vi "Fitness Core Override.vi"(8 "error in (no error)":errorcluster, 9 "Target Binary String (LSb[0] - MSb[n-1])":bool[](array[boolean]), 10 "Parent Binary String (LSb[0] - MSb[n-1])":bool[](array[boolean]), 11 "Sentence in":refnum<class "Sentence.lvclass">) -> (0 "error out":errorcluster, 2 "Fitness Score":dbl, 3 "Sentence out":refnum<class "Sentence.lvclass">)   [LabVIEW 2016, in "Sentence.lvclass"]
uses:
  Sentence.lvclass
  IChromosome/IChromosome.lvclass
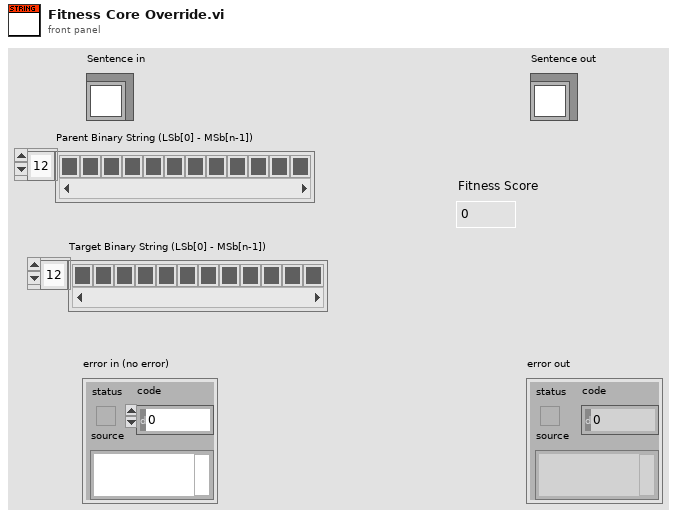
[diagram p1: front panel]
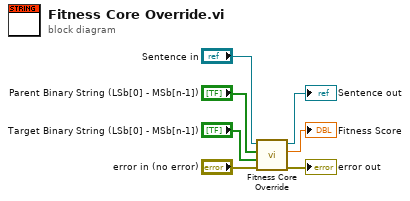
[diagram p0: block diagram]
diagram:
  n1 = call-parent "Fitness Core Override.vi"("error in (no error)"="error in (no error)", "Target Binary String (LSb[0] - MSb[n-1])"="Target Binary String (LSb[0] - MSb[n-1])", "Parent Binary String (LSb[0] - MSb[n-1])"="Parent Binary String (LSb[0] - MSb[n-1])", "IChromosome in"="Sentence in") -> ("error out"=→"error out":errorcluster, "Fitness Score"=→"Fitness Score":dbl, "IChromosome out"=→"Sentence out":refnum<class "Sentence.lvclass">)  [unwired: 5 in]
